vi "mod_Baseband PLL.vi"(0 "baseband waveform (complex)":T1={"t0"=0.0, "dt"=1.0, "Y"=[]} {"Y" format="%.3f"; "dt" format="%^.2e"; "t0" format="%.4f"}, 1 "loop filter (reverse coefficients)":dbl[](array[numeric])=[1.0, -1.0], 5 "VCO carrier frequency (Hz)":dbl, 7 "VCO initial phase (degrees)":dbl, 9 "VCO gain (degrees/V)":dbl=1.0 format="%#_6p", 11 "error in (no error)":errorcluster, 12 "loop filter (forward coefficients)":dbl[](array[numeric])=[1.05, -0.95], 13 "reset ?(T)":bool=TRUE) -> (4 "VCO phase (degrees)":dbl[](array[numeric]), 6 "phase error (degrees)":dbl[](array[numeric]), 8 "estimated carrier frequency (Hz)":dbl, 10 "estimated initial phase (degrees)":dbl, 15 "error out":errorcluster)   [LabVIEW 2020, in "niAMT.lvlib"]
uses:
  <vilib>/addons/Modulation/niAMT.lvlib
  <vilib>/addons/Modulation/Analog/controls/Complex Data Waveform.ctl
  <vilib>/Analysis/NI_AALPro.lvlib
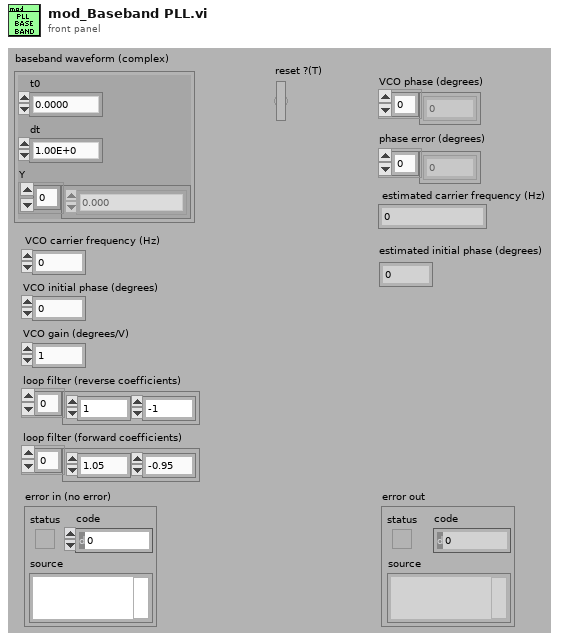
[diagram p1: front panel]
types:
  T1 = typedef "niAMT.lvlib/Complex Data Waveform.ctl" = cluster{"t0":dbl, "dt":dbl, "Y":cdb[]}
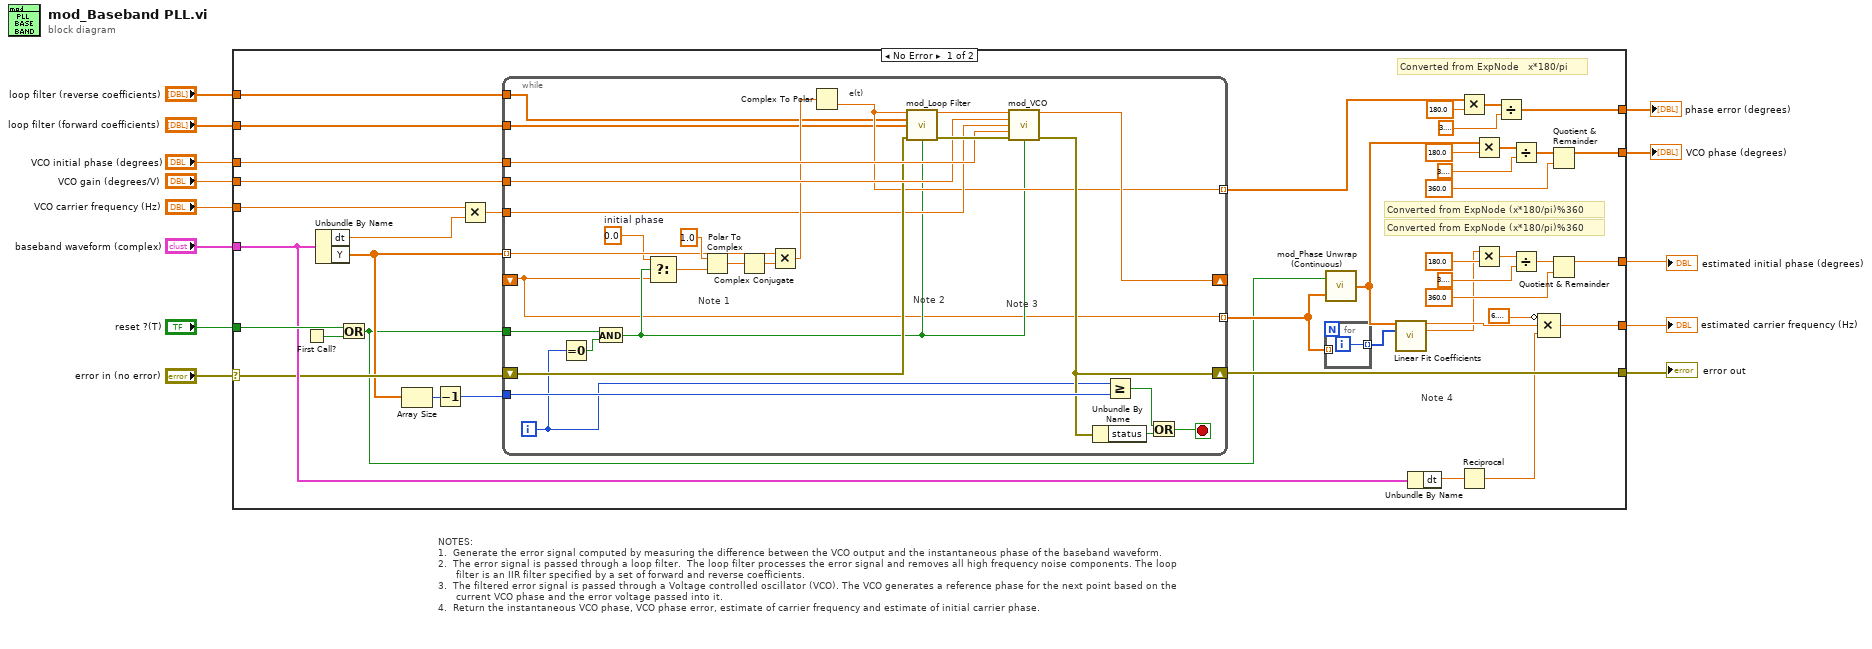
[diagram p0: block diagram]
diagram:
  # "NOTES:\n1.  Generate the error signal computed by measuring the difference between the VCO output and the instantaneous phase of the baseband waveform.\n2.  The error signal is passed through a loop filter.  The loop filter processes the error signal and removes all high frequency noise components. The loop\n      filter is an IIR filter specified by a set of forward and reverse coefficients.\n3.  The filtered error signal is passed through a Voltage controlled oscillator (VCO). The VCO generates a reference phase for the next point based on the\n      current VCO phase and the error voltage passed into it.\n4.  Return the instantaneous VCO phase, VCO phase error, estimate of carrier frequency and estimate of initial carrier phase."
  n1 = case shown="No Error" "error in (no error)" {
    selector: "error in (no error)" -> [w49 w84]
    tunnel: "reset ?(T)" -> [w54 _]
    tunnel: "baseband waveform (complex)" -> [w52 _]
    tunnel: [w48 w84] -> w10
    tunnel: "loop filter (reverse coefficients)" -> [w38 _]
    tunnel: "loop filter (forward coefficients)" -> [w37 _]
    tunnel: "VCO gain (degrees/V)" -> [w36 _]
    tunnel: "VCO carrier frequency (Hz)" -> [w35 _]
    tunnel: "VCO initial phase (degrees)" -> [w34 _]
    tunnel: [w21 _] -> w4
    tunnel: [w28 _] -> w3
    tunnel: [w14 _] -> w2
    tunnel: [w33 _] -> w1
    frame No Error {
      # "Converted from ExpNode (x*180/pi)%360"
      # "Converted from ExpNode (x*180/pi)%360"
      # "Converted from ExpNode\t\t\tx*180/pi"
      # "Note 4"
      n2 = First Call?() -> (First Call?: T/F=w50:bool)
      n3 = Unbundle By Name(w52) -> ("dt"=w55:dbl, "Y"=w47:cdb[])
      n4 = Or(x=w54, y=w50) -> (x .or. y?=w42:bool)
      n5 = Array Size(array=w47) -> (size(s)=w46:i32)
      n6 = Decrement(x=w46) -> (x-1=w45:i32)
      n7 = Multiply(x=w35, y=w55) -> (x*y=w43:dbl)
      n8 = while {
        shift-right: [w76] -> _
        shift-left: _ -> [w59]
        tunnel: [w59] -> w44 mode=indexing
        tunnel: w47 -> [w80] mode=indexing
        tunnel: w43 -> [w67]
        tunnel: w34 -> [w78]
        tunnel: w36 -> [w77]
        shift-right: [w71] -> w48
        shift-left: w49 -> [w75]
        tunnel: w45 -> [w73]
        tunnel: [w65] -> w29 mode=indexing
        tunnel: w37 -> [w57]
        tunnel: w42 -> [w62]
        tunnel: w38 -> [w56]
        i -> [w64]
        stop <- w69 stop-if-true
        w60 = 0.0  # initial phase
        # "Note 3"
        # "Note 2"
        # "Note 1"
        # "e(t)"
        n9 = Equal To 0?(x=w64) -> (x = 0?=w63:bool)
        n10 = And(x=w62, y=w63) -> (x .and. y?=w61:bool)
        n11 = Select(t=w60, s=w61, f=w59) -> (s? t:f=w58:dbl)
        n12 = Polar To Complex(1:w58, 2:1.0 ("r")) -> (0:w66:cdb)
        n13 = Complex Conjugate(1:w66) -> (0:w81:cdb)
        n14 = Multiply(x=w80, y=w81) -> (x*y=w74:cdb)
        n15 = Complex To Polar(r * e^(i*theta)=w74) -> (theta=w65:dbl)  [unwired: 1 out]
        n16 = call <vilib>:"mod_Loop Filter.vi"("x(n)"=w65, "reverse coefficients"=w56, "forward coefficients"=w57, "error in (no error)"=w75, "reset ? (T)"=w61) -> ("y(n)"=w68:dbl, "error out"=w79:errorcluster)  [unwired: 9 out]
        n17 = call <vilib>:"mod_VCO.vi"("e(n)"=w68, "gain (kf)"=w77, "carrier frequency (normalized)"=w67, "initial phase (degrees)"=w78, "error in (no error)"=w79, "reset ?(T)"=w61) -> ("theta(n)"=w76:dbl, "error out"=w71:errorcluster)  [unwired: 8 out]
        n18 = Unbundle By Name(w71) -> ("status"=w70:bool)
        n19 = Greater Or Equal?(x=w64, y=w73) -> (x >= y?=w72:bool)
        n20 = Or(x=w72, y=w70) -> (x .or. y?=w69:bool)
      }
      n21 = for {
        tunnel: [w83] -> w53 mode=indexing
        tunnel: w44 -> [_] mode=indexing
        i -> [w83]
      }
      n22 = call <vilib>:"mod_Phase Unwrap (Continuous).vi"("Input Signal"=w44, "Reset"=w42) -> ("Phase Unwrapped"=w22:dbl[])
      n23 = call <vilib>:"Linear Fit Coefficients.vi"("Y"=w22, "X"=w53) -> ("slope"=w41:dbl, "intercept"=w15:dbl)  [unwired: 3 in, 9 out]
      n24 = Unbundle By Name(w52) -> ("dt"=w51:dbl)
      n25 = Multiply(x=w29, y=180.0) -> (x*y=w31:dbl[])
      n26 = Reciprocal(x=w51) -> (1/x=w40:dbl)
      n27 = Multiply(x=w22, y=180.0) -> (x*y=w26:dbl[])
      n28 = Multiply(x=w15, y=180.0) -> (x*y=w16:dbl)
      n29 = Divide(x=w31, y=3.141592653589793) -> (x/y=w28:dbl[])
      n30 = Divide(x=w26, y=3.141592653589793) -> (x/y=w24:dbl[])
      n31 = Divide(x=w16, y=3.141592653589793) -> (x/y=w19:dbl)
      n32 = Compound Arithmetic op=MULTIPLY(invert 6.283185307179586, w41, w40) -> (w33:dbl)
      n33 = Quotient & Remainder(x=w24, y=360.0) -> (x-y*floor(x/y)=w21:dbl[])  [unwired: 1 out]
      n34 = Quotient & Remainder(x=w19, y=360.0) -> (x-y*floor(x/y)=w14:dbl)  [unwired: 1 out]
    }
    frame Error {
    }
  }
  "error out" <- w10
  "VCO phase (degrees)" <- w4
  "phase error (degrees)" <- w3
  "estimated initial phase (degrees)" <- w2
  "estimated carrier frequency (Hz)" <- w1
